vi "Init.vi"(8 "error in (no error)":errorcluster, 11 "Cursor in":refnum<class "Cursor.lvclass">) -> (0 "error out":errorcluster, 3 "Cursor out":refnum<class "Cursor.lvclass">)   [LabVIEW 2019, in "RT_Game.lvlib" / "Cursor.lvclass"]
uses:
  Cursor.lvclass
  C:/Users/FreshBob/Dropbox/VIs/myRIO_GameConsole/RT/RT_Game/RT_Sprite/RT_Sprite.lvclass
  C:/Users/FreshBob/Dropbox/VIs/myRIO_GameConsole/RT/RT_Game/GameObject/GameObject.lvclass
  Cursor.lvclass/Cursor.ctl
  RT_Sprite/RT_Sprite.lvclass
  GameObject/GameObject.lvclass
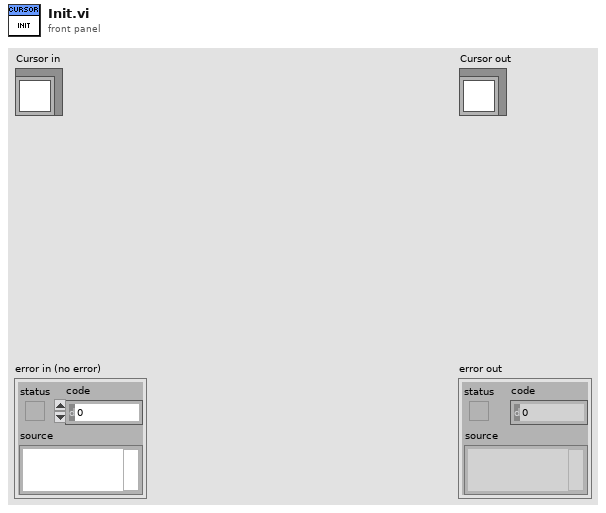
[diagram p1: front panel]
types:
  T1 = typedef "RT_Game.lvlib/Engine.lvclass/Coordinate.ctl" = cluster{"x":dbl, "y":dbl}
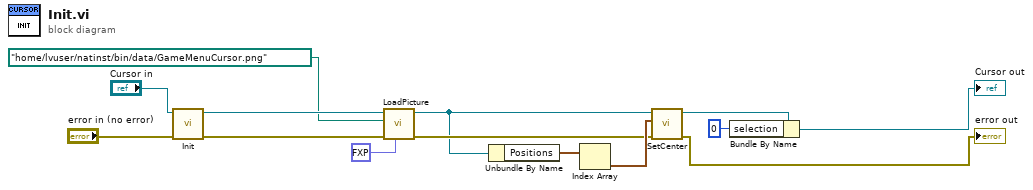
[diagram p0: block diagram]
diagram:
  n1 = call-parent "Init.vi"("error in (no error)"="error in (no error)", "RT_Sprite in"="Cursor in") -> ("error out"=w14:errorcluster, "RT_Sprite out"=w4:refnum<class "Cursor.lvclass">)  [unwired: 8 in]
  n2 = call "LoadPicture.vi"("Transparent Color"=fxp<+,3,3> 2.0, "error in (no error)"=w14, "Picture Path"=path "/home/lvuser/natinst/bin/data/GameMenuCursor.png", "RT_Sprite in"=w4) -> ("error out"=w5:errorcluster, "RT_Sprite out"=w3:refnum<class "Cursor.lvclass">)  [unwired: 6 in]
  n3 = Unbundle By Name(w3) -> ("Positions"=w9:T1[])
  n4 = Index Array(array=w9) -> (element=w8:T1)  [unwired: 1 in]
  n5 = call "SetCenter.vi"("error in (no error)"=w5, "center_position"=w8, "GameObject in"=w3) -> ("error out"=→"error out":errorcluster, "GameObject out"=w10:refnum<class "Cursor.lvclass">)  [unwired: 7 in]
  n6 = Bundle By Name(cluster=w10, "selection"=i16 0) -> (→"Cursor out":refnum<class "Cursor.lvclass">)
